vi "READ - File & Channels INFO.vi"(0 "reference in":refnum<class "HeadAcousticHDF.lvclass">, 5 "error in (no error)":errorcluster, 7 "Path - READ":path) -> (13 "Channel info":T1(array[cluster]), 14 "reference out":refnum<class "HeadAcousticHDF.lvclass">, 19 "error out":errorcluster)   [LabVIEW 2020, in "HeadAcousticHDF.lvclass"]
uses:
  HeadAcousticHDF.lvclass
  <vilib>/Platform/storage/utility/usiProperty.ctl
  <vilib>/Platform/storage/utility/usiObjectType.ctl
  <vilib>/express/express shared/ex_EditUserDefinedProperties/usiDataType.ctl
  <vilib>/Platform/storage/lvStorage.llb/_openStorageWithRootAutoDetect.vi
  <vilib>/Platform/storage/lvStorage.llb/xStorage/xStorageSupp/ErrorOut.vi
  <vilib>/Platform/storage/Storage.llb/__loadPropString.vi
  <vilib>/Platform/storage/Storage.llb/__loadPropTime.vi
  <vilib>/Platform/storage/Storage.llb/__loadPropRefList.vi
  <vilib>/Platform/storage/Storage.llb/Get Property (String).vi
  <vilib>/Platform/storage/Storage.llb/Get Property (I32).vi
  <vilib>/Platform/storage/Storage.llb/Get Property (DBL).vi
  <vilib>/Platform/storage/Storage.llb/Get Object Info.vi
  <vilib>/Platform/storage/Storage.llb/__closeStorageFromObject.vi
  <vilib>/Platform/storage/lvStorage.llb/xStorage/Open Data Storage/Open Data Storage.xnode
  <vilib>/Platform/storage/lvStorage.llb/xStorage/Get Properties/Get Properties.xnode
  <vilib>/Platform/storage/lvStorage.llb/xStorage/Close Data Storage/Close Data Storage.xnode
  API/Generic Utilities_class/Generic Utilities.lvclass
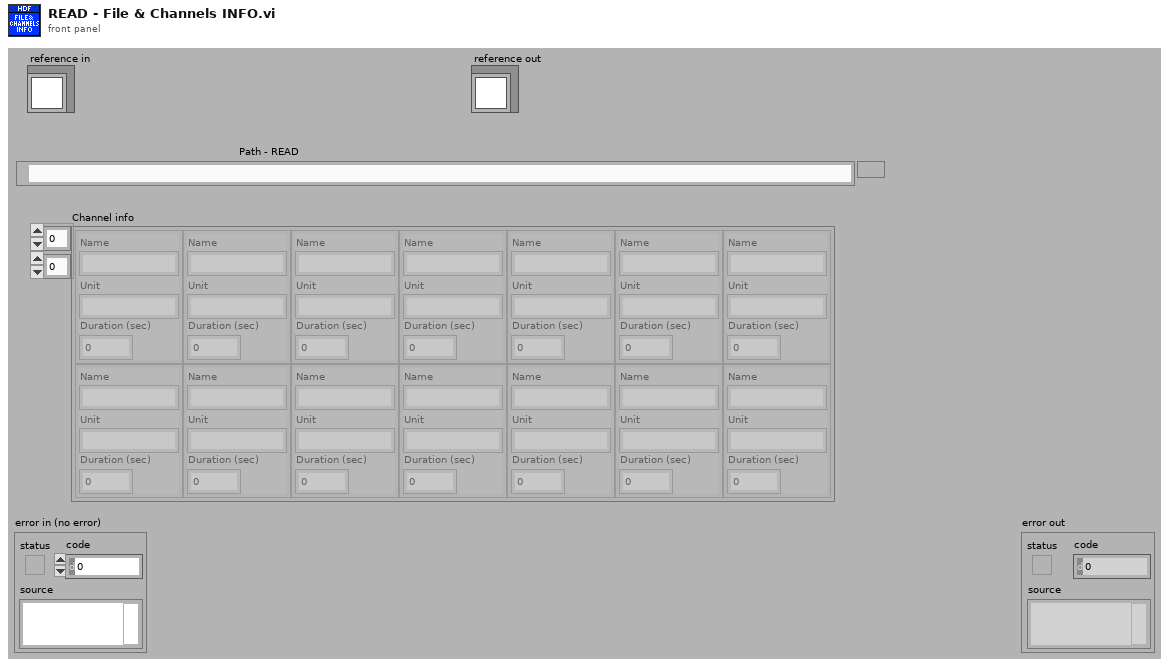
[diagram p1: front panel]
types:
  T1 = cluster{"Name":string, "Unit":string, "Duration (sec)":dbl}[][]
  T2 = typedef "usiProperty.ctl" = cluster{"object type":T3, "property name":string, "data type":T4}
  T3 = typedef "usiObjectType.ctl" = enum16{"File", "Channel Group", "Channel", "Unknown"}
  T4 = typedef "usiDataType.ctl" = enum16{"eNoTypeUsi", "eInt8Usi", "eInt16Usi", "eInt32Usi", "eInt64Usi", "eUInt8Usi", "eUInt16Usi", "eUInt32Usi", "eUInt64Usi", "eFloat32Usi", "eFloat64Usi", "- 0", "- 1", "- 2", "- 3", "- 4", "- 5", "- 6", "- 7", "- 8", "- 9", "eString8Usi", "eString16Usi", "eStringUsi", "eEnumUsi", "- 10", "- 11", "- 12", "- 13", "- 14", "eTimeUsi", "- 15", "- 16", "- 17", "- 18", "- 19", "- 20", "- 21", "- 22", "- 23", "eInstanceUsi", "eStoreUsi"}
  T5 = enum16{"open", "open or create", "create or replace", "create", "open (read only)"}
  T6 = enum16{"UPDATE", "READ", "QUERY", "CREATE CHILD", "CREATE", "CONNECT", "DISCONNECT"}
  T7 = typedef "HeadAcousticHDF.lvclass/ObjectAttributesRef.ctl" = refnum<data-value>
  T8 = typedef "HeadAcousticHDF.lvclass/ObjectAttributes.ctl" = cluster{"Time Data":refnum<class "GSwFormDSP.lvclass">, "Data Plugin Name":string, "Additional Data Plugin Name":string, "New Time Data Obj?":bool}
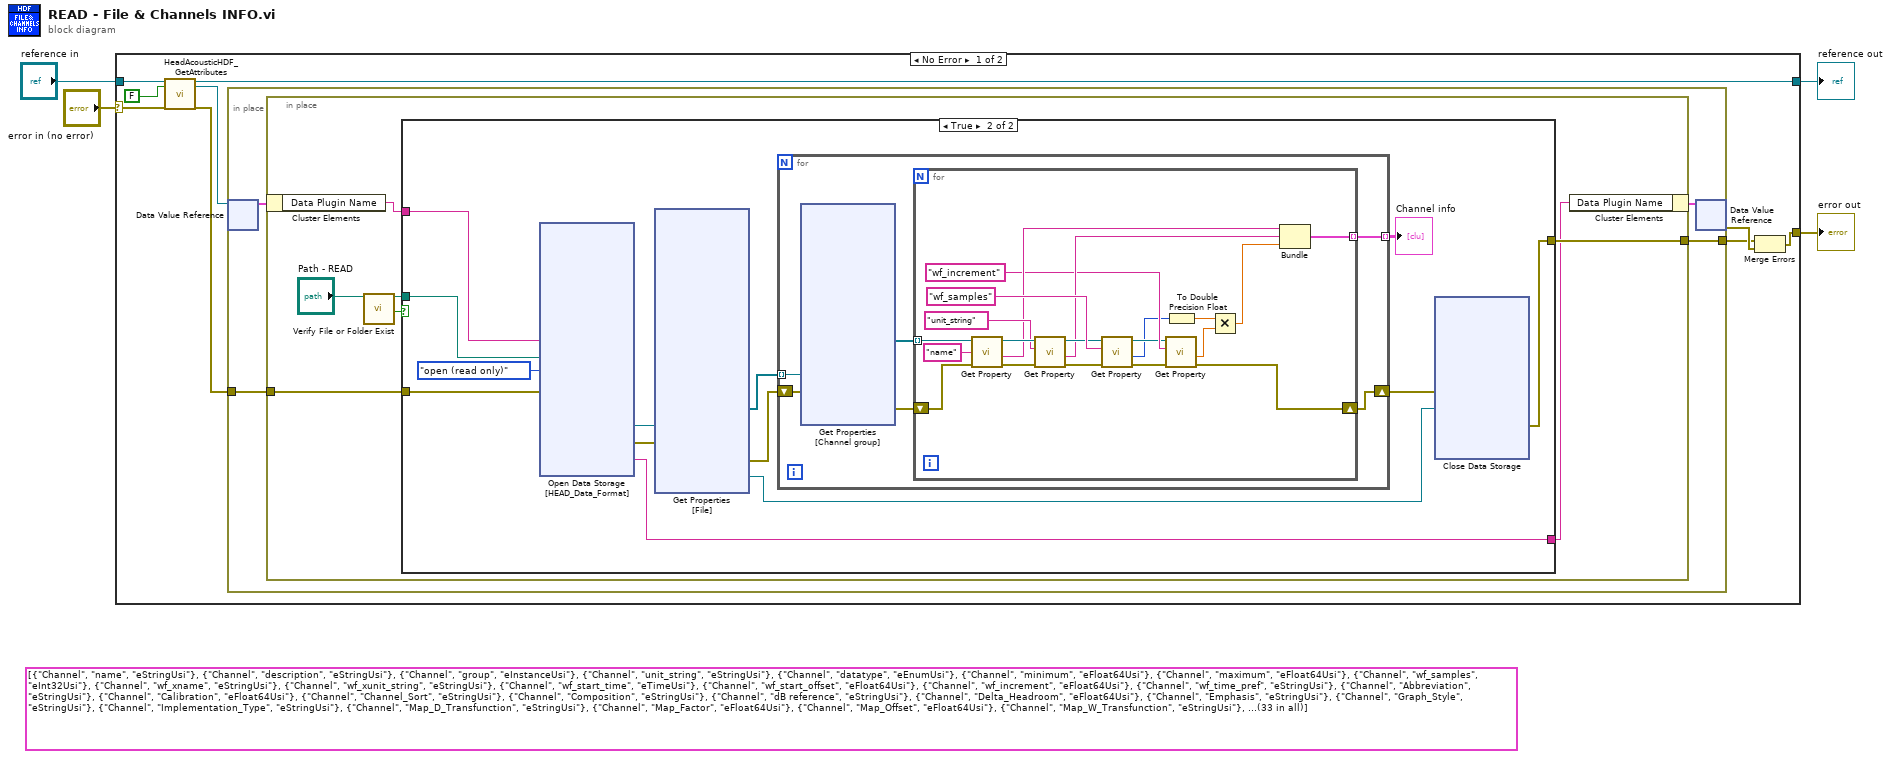
[diagram p0: block diagram]
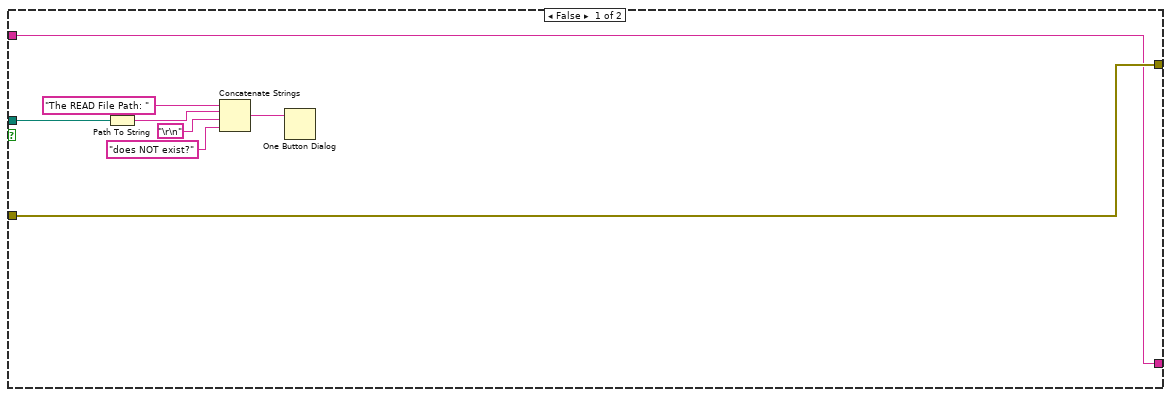
[diagram p2: hidden frame]
diagram:
  (unwired) T2[] [{"object type"=enum."Channel", "property name"="name", "data type"=enum."eStringUsi"}, {"object type"=enum."Channel", "property name"="description", "data type"=enum."eStringUsi"}, {"object type"=enum."Channel", "property name"="group", "data type"=enum."eInstanceUsi"}, {"object type"=enum."Channel", "property name"="unit_string", "data type"=enum."eStringUsi"}, {"object type"=enum."Channel", "property name"="datatype", "data type"=enum."eEnumUsi"}, {"object type"=enum."Channel", "property name"="minimum", "data type"=enum."eFloat64Usi"}, {"object type"=enum."Channel", "property name"="maximum", "data type"=enum."eFloat64Usi"}, {"object type"=enum."Channel", "property name"="wf_samples", "data type"=enum."eInt32Usi"}, {"object type"=enum."Channel", "property name"="wf_xname", "data type"=enum."eStringUsi"}, {"object type"=enum."Channel", "property name"="wf_xunit_string", "data type"=enum."eStringUsi"}, {"object type"=enum."Channel", "property name"="wf_start_time", "data type"=enum."eTimeUsi"}, {"object type"=enum."Channel", "property name"="wf_start_offset", "data type"=enum."eFloat64Usi"}, {"object type"=enum."Channel", "property name"="wf_increment", "data type"=enum."eFloat64Usi"}, {"object type"=enum."Channel", "property name"="wf_time_pref", "data type"=enum."eStringUsi"}, {"object type"=enum."Channel", "property name"="Abbreviation", "data type"=enum."eStringUsi"}, {"object type"=enum."Channel", "property name"="Calibration", "data type"=enum."eFloat64Usi"}, {"object type"=enum."Channel", "property name"="Channel_Sort", "data type"=enum."eStringUsi"}, {"object type"=enum."Channel", "property name"="Composition", "data type"=enum."eStringUsi"}, {"object type"=enum."Channel", "property name"="dB reference", "data type"=enum."eStringUsi"}, {"object type"=enum."Channel", "property name"="Delta_Headroom", "data type"=enum."eFloat64Usi"}, {"object type"=enum."Channel", "property name"="Emphasis", "data type"=enum."eStringUsi"}, {"object type"=enum."Channel", "property name"="Graph_Style", "data type"=enum."eStringUsi"}, {"object type"=enum."Channel", "property name"="Implementation_Type", "data type"=enum."eStringUsi"}, {"object type"=enum."Channel", "property name"="Map_D_Transfunction", "data type"=enum."eStringUsi"}, {"object type"=enum."Channel", "property name"="Map_Factor", "data type"=enum."eFloat64Usi"}, {"object type"=enum."Channel", "property name"="Map_Offset", "data type"=enum."eFloat64Usi"}, {"object type"=enum."Channel", "property name"="Map_W_Transfunction", "data type"=enum."eStringUsi"}, {"object type"=enum."Channel", "property name"="Moniker", "data type"=enum."eStringUsi"}, {"object type"=enum."Channel", "property name"="Physical_Channel", "data type"=enum."eInt32Usi"}, {"object type"=enum."Channel", "property name"="Physical_Quantity", "data type"=enum."eStringUsi"}, {"object type"=enum."Channel", "property name"="Quantisation_Function", "data type"=enum."eStringUsi"}, {"object type"=enum."Channel", "property name"="range offset", "data type"=enum."eStringUsi"}, {"object type"=enum."Channel", "property name"="Title", "data type"=enum."eStringUsi"}] ("properties")
  n1 = case shown="No Error" "error in (no error)" {
    selector: "error in (no error)" -> [w8 w135]
    tunnel: [w13 w135] -> w3
    tunnel: [w7 w134] -> w1
    tunnel: "reference in" -> [w10 w134]
    frame No Error {
      n2 = call "HeadAcousticHDF_GetAttributes.vi"("reference in"=w10, "return data? (T)"=FALSE, "error in (no error)"=w8) -> ("reference out"=w7:refnum<class "HeadAcousticHDF.lvclass">, "attributes ref"=w6:T7, "error out"=w5:errorcluster)  [unwired: 13 in, 1 out]
      n3 = in-place {
        in-place-border: [w14] -> w11
        in-place-border: w5 -> [w15]
        n4 = in-place-dvr #1(w6) -> (w16:T8)  [unwired: 1 out]
        n5 = in-place {
          in-place-border: w15 -> [w21]
          in-place-border: [w20] -> w14
          n6 = in-place-cluster #2(w16) -> ("Data Plugin Name"=w19:string)
          n7 = call "Verify File or Folder Exist.vi"("path"="Path - READ") -> ("dup path"=w24:path, "file or folder exists?"=w23:bool)  [unwired: 16 in, 1 out]
          n8 = case shown="True" w23 {
            tunnel: w24 -> [w31 w44]
            tunnel: w21 -> [w32 w42]
            tunnel: [w32 w37] -> w20
            tunnel: w19 -> [w25 w45]
            tunnel: [w25 w41] -> w18
            frame False {
              n9 = Path To String(path=w31) -> (string=w29:string)
              n10 = Concatenate Strings("The READ File Path: ", w29, "\r\n", "does NOT exist?") -> (w26:string)
              n11 = One Button Dialog(message=w26) -> ()  [unwired: 1 in, 1 out]
            }
            frame True {
              n12 = xnode "Open Data Storage\n[HEAD_Data_Format]"("DataPlugin name"=w45, "file path"=w44, "function (open:0)"=T5."open (read only)", "error in (no error)"=w42) -> ("storage refnum (file)"=w40:refnum<k20>, "error out"=w39:errorcluster, "DataPlugin name out"=w41:string)  [unwired: 1 in]
              n13 = xnode "Get Properties\n[File]"("storage refnum (file)"=w40, "error in"=w39) -> ("storage refnums (channel group)"=w34:refnum<k20>[], "error out"=w36:errorcluster, "storage refnum (file) out"=w38:refnum<k20>)  [unwired: 5 out]
              n14 = for {
                shift-right: [w49] -> w35
                shift-left: w36 -> [w51]
                tunnel: w34 -> [w47] mode=indexing
                tunnel: [w46] -> w33 mode=indexing
                n15 = xnode "Get Properties\n[Channel group]"("storage refnum (channel group)"=w47, "error in"=w51) -> ("storage refnums (channel)"=w48:refnum<k20>[], "error out"=w50:errorcluster)  [unwired: 3 out]
                n16 = for {
                  shift-right: [w54] -> w49
                  shift-left: w50 -> [w69]
                  tunnel: w48 -> [w71] mode=indexing
                  tunnel: [w52] -> w46 mode=indexing
                  n17 = call-poly <vilib>:"Get Property.vi"("error in (no error)"=w69, "Property name"="name" ("property name"), "storage refnum"=w71) -> ("error out"=w67:errorcluster, "Value"=w62:string, "storage refnum out"=w68:refnum<k20>)  [unwired: 6 in]
                  n18 = call-poly <vilib>:"Get Property.vi"("error in (no error)"=w67, "Property name"="unit_string" ("property name"), "storage refnum"=w68) -> ("error out"=w63:errorcluster, "Value"=w61:string, "storage refnum out"=w64:refnum<k20>)  [unwired: 6 in]
                  n19 = call-poly <vilib>:"Get Property.vi"("error in (no error)"=w63, "Property name"="wf_samples" ("property name"), "storage refnum"=w64) -> ("error out"=w58:errorcluster, "Value"=w57:i32, "storage refnum out"=w59:refnum<k20>)  [unwired: 6 in]
                  n20 = call-poly <vilib>:"Get Property.vi"("error in (no error)"=w58, "Property name"="wf_increment" ("property name"), "storage refnum"=w59) -> ("error out"=w54:errorcluster, "Value"=w55:dbl)  [unwired: 6 in, 1 out]
                  n21 = To Double Precision Float(number=w57) -> (double precision float=w56:dbl)
                  n22 = Multiply(x=w56, y=w55) -> (x*y=w53:dbl)
                  n23 = Bundle("Value"=w62, "Value"=w61, w53) -> (w52:cluster{"Value":string, "Value":string, dbl})  [unwired: 1 in]
                }
              }
              "Channel info" <- w33
              n24 = xnode "Close Data Storage\n"("error in (no error)"=w35, "storage refnum (file)"=w38) -> ("error out"=w37:errorcluster)  [unwired: 1 out]
            }
          }
          n25 = in-place-cluster #2("Data Plugin Name"=w18) -> (w17:T8)
        }
        n26 = in-place-dvr #1(w17) -> (w12:errorcluster)  [unwired: 1 out]
      }
      n27 = Merge Errors(w11, w12) -> (w13:errorcluster)
    }
    frame Error {
    }
  }
  "error out" <- w3
  "reference out" <- w1
